vi "Write message.vi"(8 "error in (no error)":errorcluster, 10 "message":string, 11 "MB_TCP in":refnum<class "MB_TCP.lvclass">) -> (0 "error out":errorcluster, 3 "MB_TCP out":refnum<class "MB_TCP.lvclass">)   [LabVIEW 2019]
uses:
  MB_TCP.lvclass
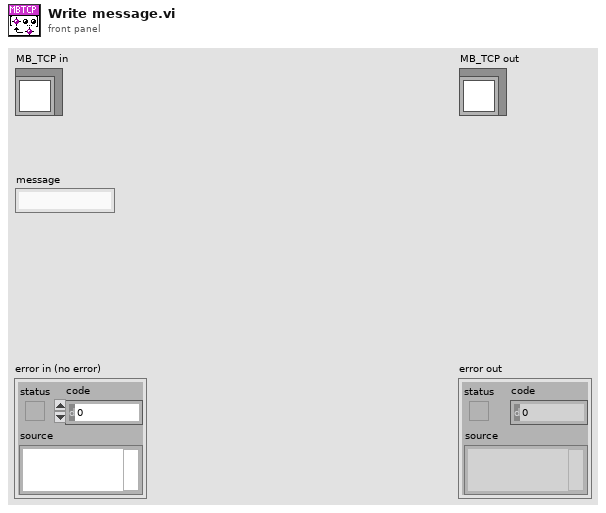
[diagram p1: front panel]
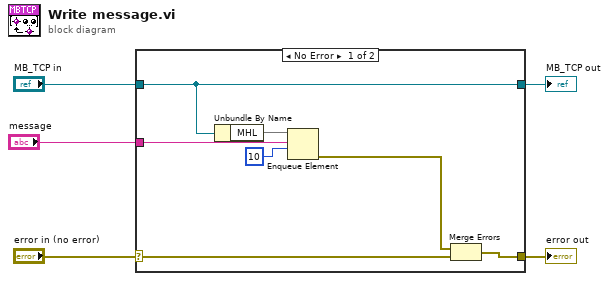
[diagram p0: block diagram]
diagram:
  n1 = case shown="No Error" "error in (no error)" {
    selector: "error in (no error)" -> [w7 w13]
    tunnel: [w6 w13] -> w4
    tunnel: [w9 w14] -> w2
    tunnel: "MB_TCP in" -> [w9 w14]
    tunnel: "message" -> [w10 _]
    frame No Error {
      n2 = Unbundle By Name(w9) -> ("MHL"=w12)
      n3 = Enqueue Element(queue=w12, element=w10, timeout in ms (-1)=10) -> (error out=w8:errorcluster)  [unwired: 1 in, 2 out]
      n4 = Merge Errors(w8, w7) -> (w6:errorcluster)
    }
    frame Error {
    }
  }
  "error out" <- w4
  "MB_TCP out" <- w2
